vi "Nuclei - sideways pull.vi"() -> ()   [LabVIEW 2010]
uses:
  <vilib>/Utility/error.llb/DialogType.ctl
  <vilib>/DAQmx/read.llb/DAQmx Read (Analog 1D DBL NChan 1Samp).vi
  <vilib>/DAQmx/write.llb/DAQmx Write (Analog DBL 1Chan 1Samp).vi
  <vilib>/DAQmx/read.llb/DAQmx Read (Analog 1D Wfm NChan NSamp).vi
  <vilib>/DAQmx/create/channels.llb/DAQmx Create Channel (AO-Voltage-Basic).vi
  <vilib>/DAQmx/create/channels.llb/DAQmx Create Channel (AI-Voltage-Basic).vi
  <vilib>/DAQmx/configure/timing.llb/DAQmx Timing (Sample Clock).vi
  <vilib>/Utility/inputDevices.llb/keyboardAcquire.vi
  <vilib>/daqmx/miscellaneous.llb/DAQmx Fill In Error Info.vi
  <vilib>/Utility/file.llb/Write To Spreadsheet File (DBL).vi
  Program Files/National Instruments/LabVIEW 2010/resource/objmgr/daqmx.rc
  <vilib>/Analysis/NI_AALBase.lvlib
panel:
  out "element":cluster{dbl[], dbl[]}
  in  "Index #":i32=1
  out "Z Position":dbl
  out "Y Position":dbl
  out "X Position":dbl
  in  "Axial Pulling":T1(tab)=enum."Piezo Move"
  in  "Reset Hysteresis":bool=TRUE
  in  "Axis":u16(ring) items=["X", "Y", "Z"]
  in  "Desired Position (um)":dbl=5.0 min=0.0 max=12.0 format="%0.2f"
  out "X Position":dbl
  out "Y Position":dbl
  out "Z Position":dbl
  in  "Move Piezo":bool=TRUE
  in  "All Axis":bool
  out "Out of Piezo Range":bool
  out "XY Graph":cluster{"Y":dbl[], "Y":dbl[]}[](graph)
  out "# of Samples":i32
  in  "wait time":u32=30
  in  "Speed":dbl=3.0
  in  "stop 3":bool
  out "X Voltage":dbl
  out "XY Graph 2":cluster{dbl[], dbl[]}(graph)
  out "Waveform Graph":dbl[][](graph)
  in  "Desired Frequency 4":dbl=0.01 caption="frequency (Hz)" format="%.2f"
  in  "Save Data":bool=TRUE
  out "?":cluster{dbl[], dbl[]}(graph)
  in  "Axis":u16(ring) items=["X", "Y", "Z"]
  in  "Cycles per Buffer":dbl=1.0 format="%.2f"
  out "Total Time":dbl
  in  "Disp Slope":dbl=-19.0
  in  "Push (nm)":dbl=30.0 min=0.0 max=10.0
  in  "Pull  (nm)":dbl=30.0 min=0.0 max=10.0
  in  "Start":dbl=5.0 min=0.0 max=10.0 format="%#_7g"
  in  "Rate (Hz)":dbl=1000.0 format="%0.2f"
  in  "Manual":bool
  out "?":dbl(graph)
  out "?":dbl(graph)
  in  "Rate":dbl=200.0 caption="Input Rate (Hz)" format="%0.2f"
  in  "Set Point (QPD)":dbl=1.6
  in  "I":dbl=0.001
  in  "P":dbl=0.1
  in  "stop 4":bool caption="stop"
  in  "Axis 2":u16(ring) items=["X", "Y", "Z"]
  in  "Rate 2":dbl=200.0 caption="Input Rate (Hz)" format="%0.2f"
  in  "Axis 3":u16(ring) items=["X", "Y", "Z"]
  out "?":dbl(graph)
  out "?":dbl(graph)
  in  "Set Point (Strain Gauge)":dbl=5.0
  in  "I":dbl=0.001
  in  "P":dbl=0.1
  in  "stop 5":bool caption="stop"
  in  "?":T2(tab)
  in  "maximum volts":dbl=10.0 format="%0.2f"
  in  "minimum volts":dbl=-10.0 format="%0.2f"
  in  "# of Samples":i32=10
  out "?":waveform(dbl)[](graph)
  in  "wait time (ms)":u32=20
  in  "stop 11":bool
  in  "QPD":u16(ring)=1 items=["QPD2", "QPD1"]
  in  "Strain Gauge":bool
  out "?":waveform(dbl)[](graph)
  in  "rate (Hz)":dbl=40000.0 format="%0.2f"
  in  "# Samples  2":i32=120000
  in  "Axis":u16(ring) items=["X", "Y", "Z"]
  out "d":cluster{"Y":dbl[], "Y":dbl[]}[](graph)
  in  "fit end (Hz)":dbl=10000.0
  in  "fit start (Hz)":dbl=30.0
  in  "nbin":dbl=5000.0
  in  "nblock":dbl=100.0
  out "fc error (Hz)  2":dbl
  out "fc (Hz)":dbl
  out "Z (um)":dbl
  in  "# of Measurements":i32=3
  in  "# Samples":i32=50000
  in  "rate (Hz)   2":dbl=50000.0 format="%0.2f"
  in  "stop 2":bool
  in  "Start (um)":dbl format="%0.2f"
  in  "Finish (um)":dbl=4.0 format="%0.2f"
  in  "Step Size (um)":dbl=1.0 format="%0.2f"
  in  "wall":dbl=1.0 format="%0.2f"
  out "Waveform Chart 2":waveform(dbl)[](graph)
  out "?":cluster{"Y":dbl[], "Y":dbl[]}[](graph)
  in  "nbin":dbl=5000.0
  out "?":cluster{"Y":dbl[], "Y":dbl[]}[](graph)
  in  "Amplitude 12":dbl=0.5 caption="Amplitude (um)" format="%0.2p"
  in  "Desired Frequency 5":dbl=0.3 caption="frequency (Hz)" format="%.2f"
  in  "Center (um)":dbl=5.0 format="%0.2p"
  in  "Save Data":bool=TRUE
  in  "Waveform Type 6":T3(ring)=enum."Triangle Wave" caption="Waveform Type"
  in  "Phase":u16(ring)=1 items=["Start", "Middle", "Right End"]
  in  "Axis":u16(ring) items=["X", "Y", "Z"]
  out "?":cluster{"Y":dbl[], "Y":dbl[]}[](graph)
  in  "Axis":u16(ring) items=["X", "Y", "Z"]
  out "Displacement Slope":dbl
  out "?":cluster{"Y":dbl[], "Y":dbl[]}[](graph)
  in  "Phase":u16(ring)=1 items=["Start", "Middle", "Right End"]
  out "X Position 3":dbl
  out "Y Position 3":dbl
  in  "Amplitude 13":dbl=0.5 caption="Amplitude (um)" format="%0.2p"
  in  "Desired Frequency 6":dbl=0.3 caption="frequency (Hz)" format="%.2f"
  in  "Waveform Type 7":T3(ring)=enum."Triangle Wave" caption="Waveform Type"
  in  "Axis":u16(ring) items=["X", "Y", "Z"]
  out "Z Position   3":dbl
  in  "Z start":dbl=5.0 format="%0.2p"
  in  "Z step size":dbl=5.0 format="%0.2p"
  in  "Z finish":dbl=5.0 format="%0.2p"
  in  "Y step size":dbl=5.0 format="%0.2p"
  in  "Y finish":dbl=5.0 format="%0.2p"
  in  "Y start":dbl=5.0 format="%0.2p"
  in  "Filename":string="test"
  # "Run to reset hysteresis!\nPlaces all piezo positions to zero and resets hysteresis parameters\nDo once at the start of the day!"
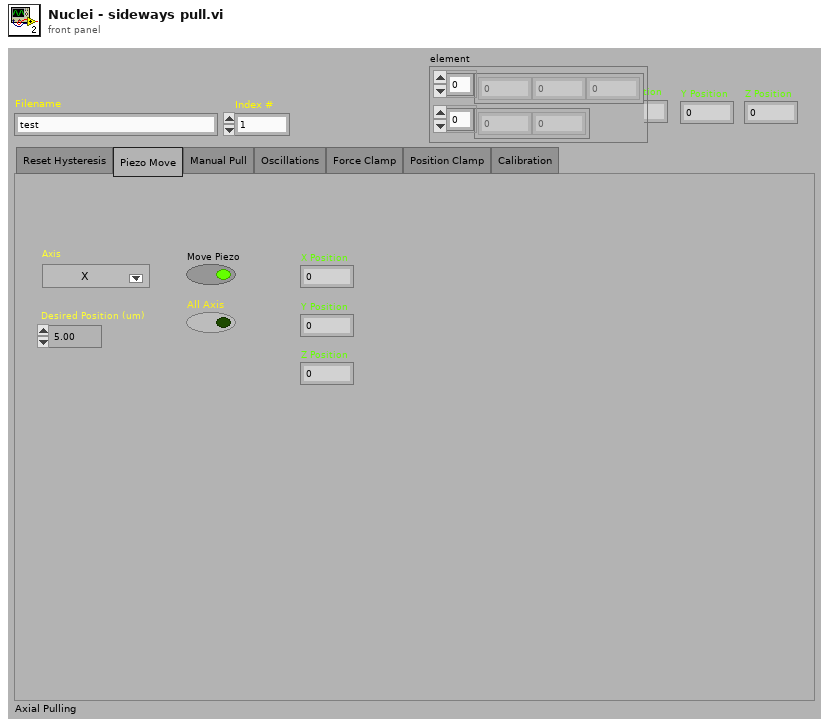
[diagram p1: front panel]
types:
  T1 = enum32{"Reset Hysteresis", "Piezo Move", "Manual Pull", "Oscillations", "Force Clamp", "Position Clamp", "Calibration"}
  T2 = enum32{"QPD", "Power Spectrum", "Axial Step Power Spectrum", "Bead Scan", "Fit Bead Scan", "3D scan"}
  T3 = enum16{"Sine Wave", "Triangle Wave", "Square Wave", "Sawtooth Wave"}
  T4 = enum16{"0", "1", "2", "3", "4", "5", "6", "7", "8", "9", "A", "B", "C", "D", "E", "F", "G", "H", "I", "J", "K", "L", "M", "N", "O", "P", "Q", "R", "S", "T", "U", "V", "W", "X", "Y", "Z", "F1", "F2", "F3", "F4", "F5", "F6", "F7", "F8", "F9", "F10", "F11", "F12", "F13", "F14", "F15", "ADD", "BACK", "BACKSLASH", "CAPITAL", "COMMA", "DECIMAL", "DELETE", "DIVIDE", "DOWN", "END", "EQUALS", "ESCAPE", "GRAVE (`)", "HOME", "INSERT", "LBRACKET", "LCONTROL", "LEFT", "L ALT", "LSHIFT", "LWIN", "MINUS", "MULTIPLY", "NEXT", "NUMLOCK", "NUMPAD_0", "NUMPAD_1", "NUMPAD_2", "NUMPAD_3", "NUMPAD_4", "NUMPAD_5", "NUMPAD_6", "NUMPAD_7", "NUMPAD_8", "NUMPAD_9", "PAUSE", "PERIOD", "PRIOR (PG UP)", "RBRACKET", "RCONTROL", "RETURN", "RIGHT", "R ALT", "RSHIFT", "RWIN", "SCROLL", "SEMICOLON", "SLASH", "SPACE", "SUBTRACT", "TAB", "UP", "ENTER (num pad)", "' (quote)"}[]
  T5 = enum16{"0", "1", "2", "3", "4", "5", "6", "7", "8", "9", "A", "B", "C", "D", "E", "F", "G", "H", "I", "J", "K", "L", "M", "N", "O", "P", "Q", "R", "S", "T", "U", "V", "W", "X", "Y", "Z", "F1", "F2", "F3", "F4", "F5", "F6", "F7", "F8", "F9", "F10", "F11", "F12", "F13", "F14", "F15", "ADD", "BACK", "BACKSLASH", "CAPITAL", "COMMA", "DECIMAL", "DELETE", "DIVIDE", "DOWN", "END", "EQUALS", "ESCAPE", "GRAVE (`)", "HOME", "INSERT", "LBRACKET", "LCONTROL", "LEFT", "L ALT", "LSHIFT", "LWIN", "MINUS", "MULTIPLY", "NEXT", "NUMLOCK", "NUMPAD_0", "NUMPAD_1", "NUMPAD_2", "NUMPAD_3", "NUMPAD_4", "NUMPAD_5", "NUMPAD_6", "NUMPAD_7", "NUMPAD_8", "NUMPAD_9", "PAUSE", "PERIOD", "PRIOR (PG UP)", "RBRACKET", "RCONTROL", "RETURN", "RIGHT", "R ALT", "RSHIFT", "RWIN", "SCROLL", "SEMICOLON", "SLASH", "SPACE", "SUBTRACT", "TAB", "UP", "ENTER (num pad)", "' (quote)"}
  T6 = typedef "DialogType.ctl" = u16
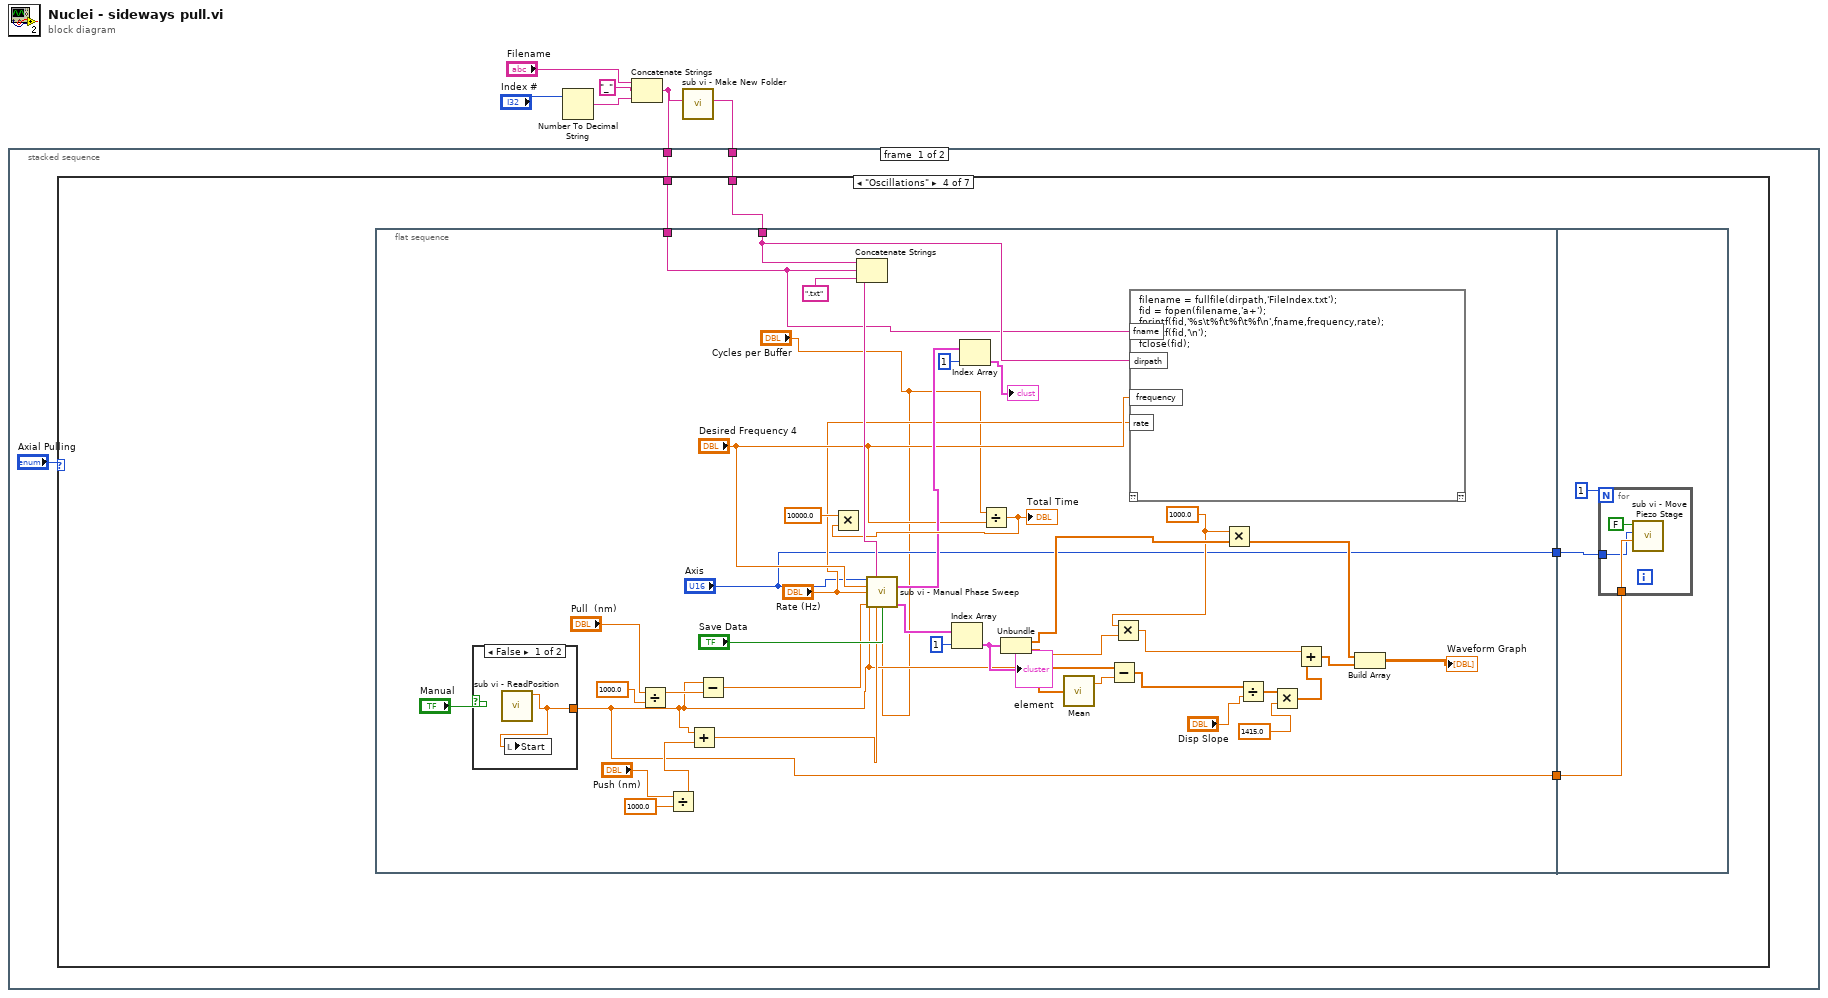
[diagram p0: block diagram]
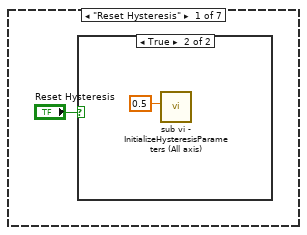
[diagram p2: hidden frame]
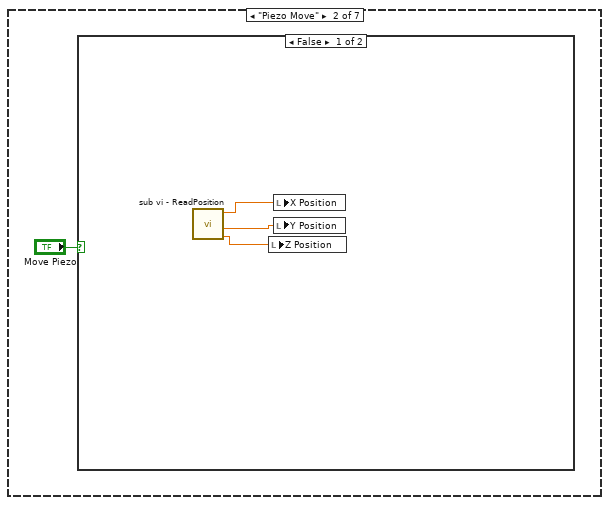
[diagram p4: hidden frame]
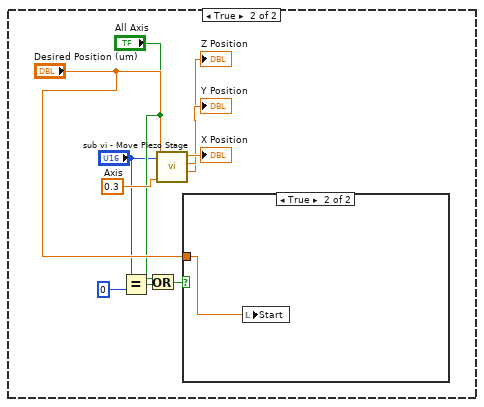
[diagram p5: hidden frame]
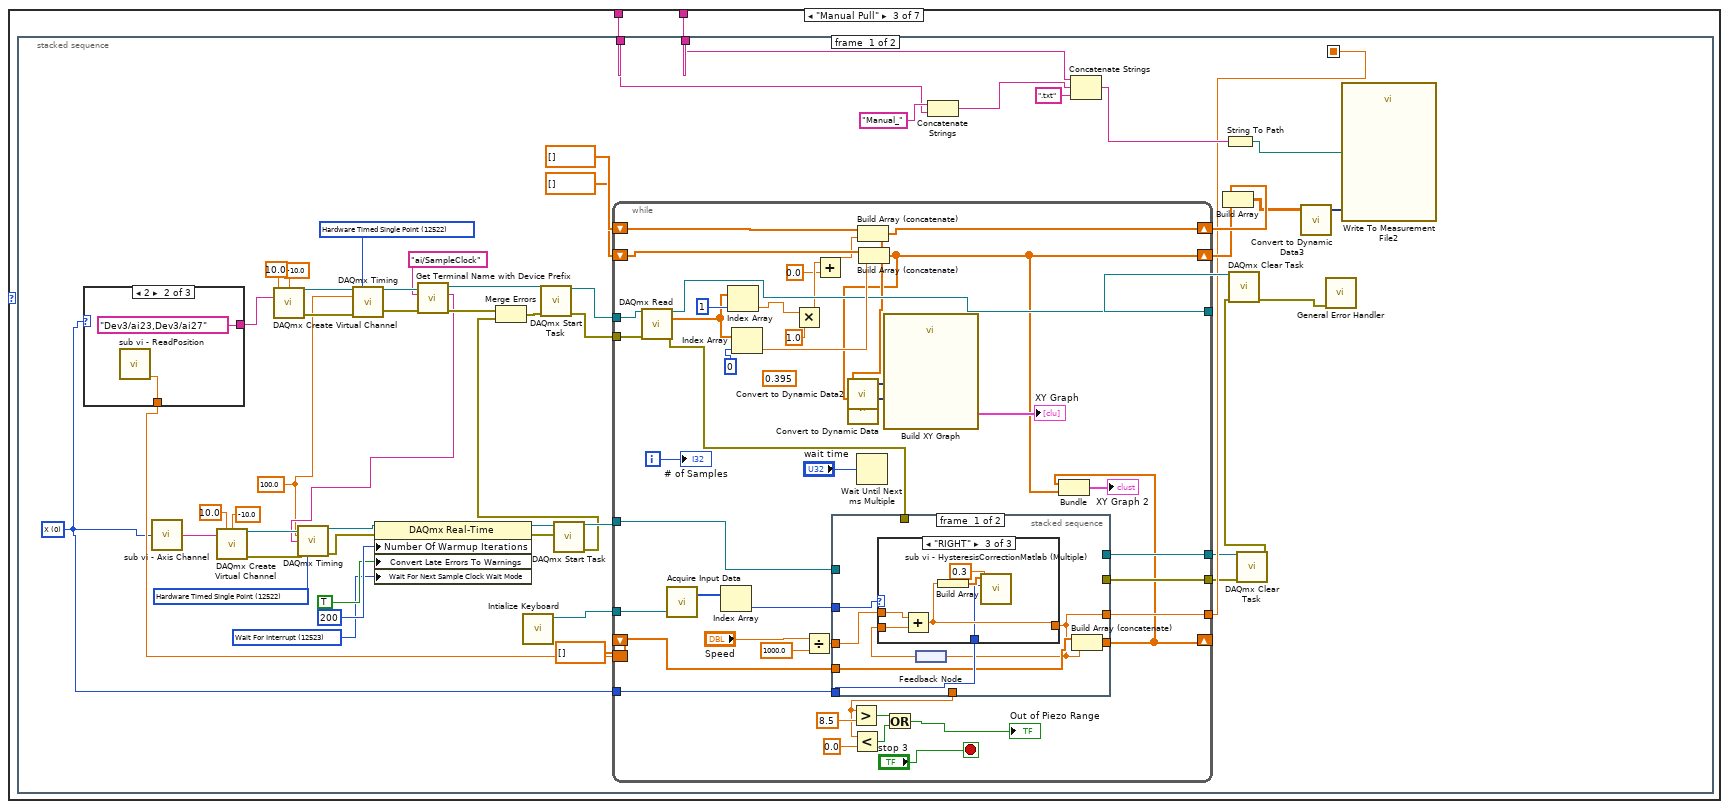
[diagram p7: hidden frame]
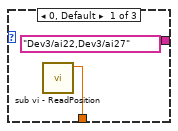
[diagram p8: hidden frame]
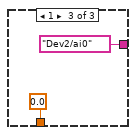
[diagram p9: hidden frame]
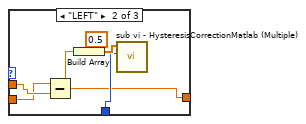
[diagram p11: hidden frame]
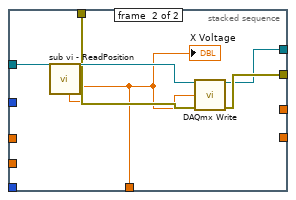
[diagram p12: hidden frame]
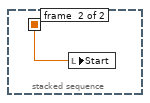
[diagram p13: hidden frame]
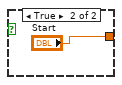
[diagram p14: hidden frame]
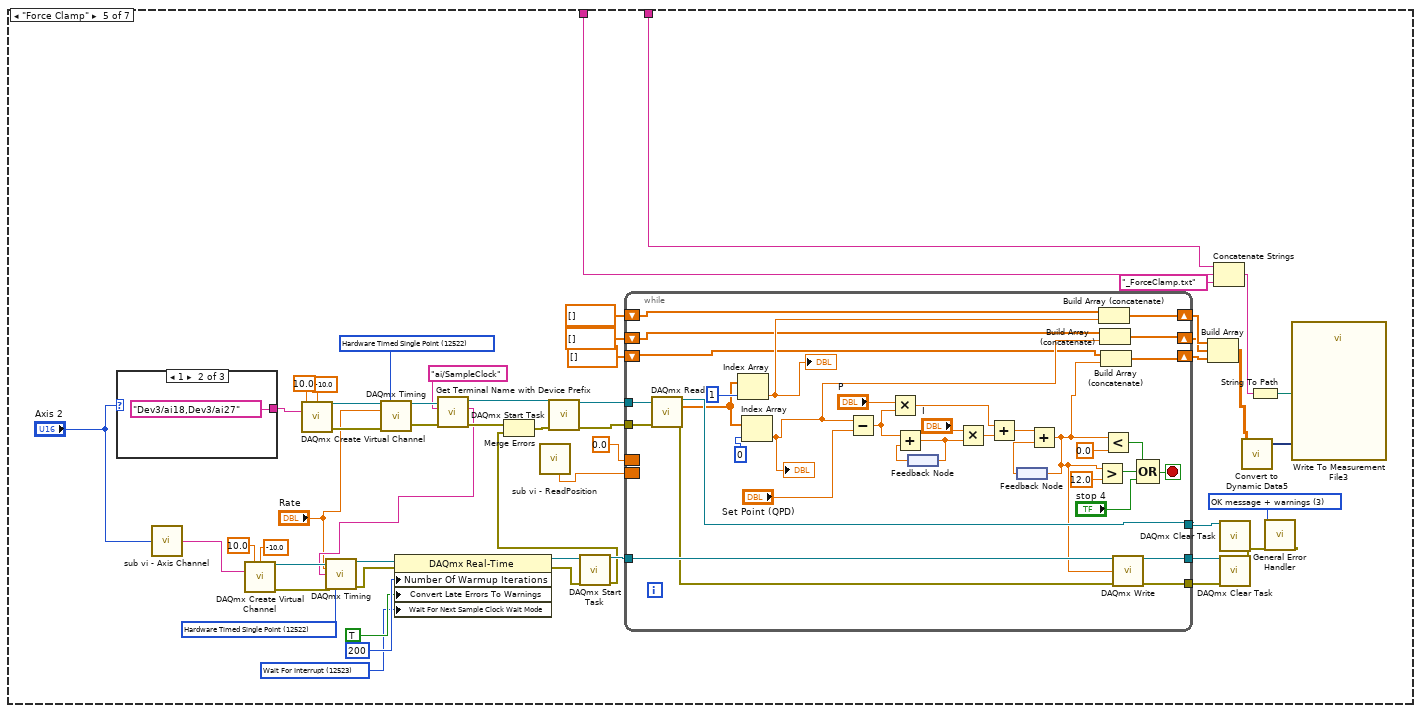
[diagram p15: hidden frame]
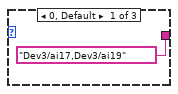
[diagram p16: hidden frame]
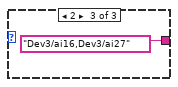
[diagram p17: hidden frame]
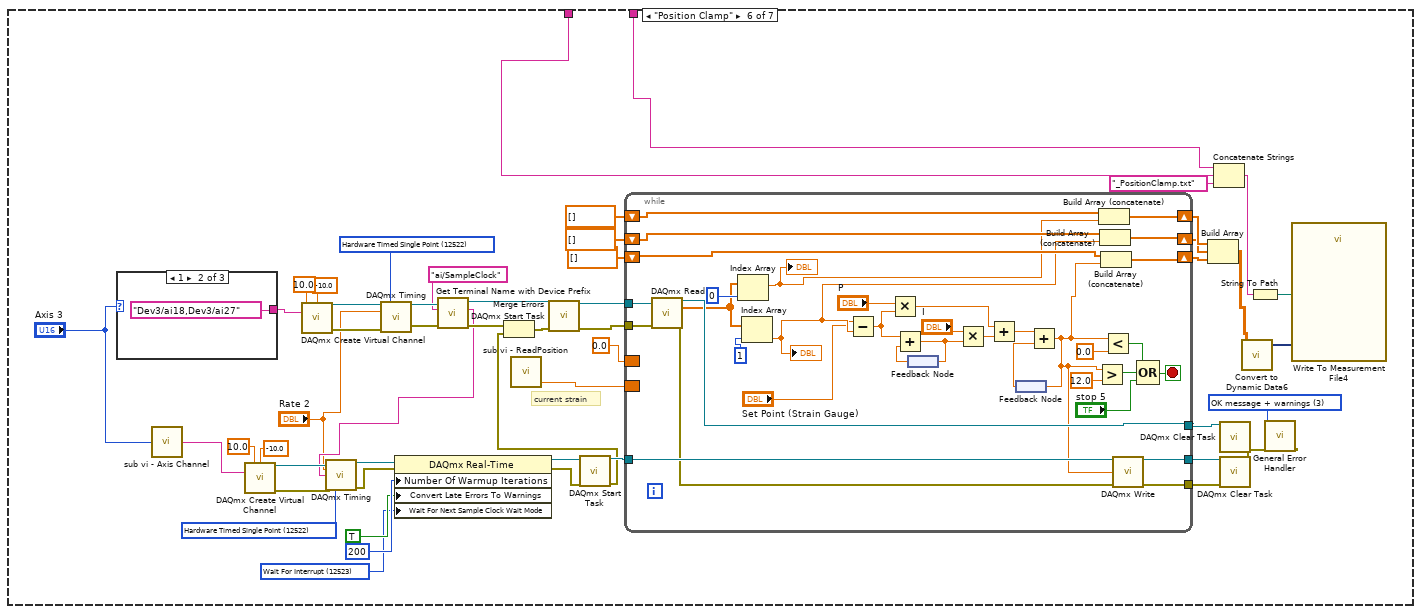
[diagram p18: hidden frame]
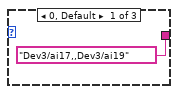
[diagram p19: hidden frame]
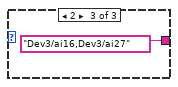
[diagram p20: hidden frame]
diagram:
  n1 = Number To Decimal String(number="Index #") -> (decimal integer string=w3:string)  [unwired: 1 out]
  n2 = Concatenate Strings("Filename", "_" ("string"), w3) -> (w1:string)
  n3 = call "sub vi - Make New Folder.vi"("folder name"=w1) -> ("directory 2"=w2:string)  [unwired: 1 in, 9 out]
  n4 = stacked-sequence {
    tunnel: w2 -> [w8 _]
    tunnel: w1 -> [w7 _]
    frame #0 {
      n5 = case shown="\"Oscillations\"" "Axial Pulling" {
        tunnel: w8 -> [_ _ w28 w160 w213 w301 w392]
        tunnel: w7 -> [_ _ w27 w159 w212 w300 w391]
        frame "Reset Hysteresis" {
          n6 = case shown="True" "Reset Hysteresis" {
            frame False {
            }
            frame True {
              n7 = call "sub vi - InitializeHysteresisParameters (All axis).vi"("frequency"=0.5) -> ()  [unwired: 11 in]
            }
          }
        }
        frame "Piezo Move" {
          n8 = case shown="False" "Move Piezo" {
            frame False {
              n9 = call "sub vi - ReadPosition.vi"() -> ("Z Position"=w13:dbl, "Y Position"=w14:dbl, "X Position"=w15:dbl)  [unwired: 9 out]
              n10 = local write "Z Position"(w13) -> ()
              n11 = local write "X Position"(w15) -> ()
              n12 = local write "Y Position"(w14) -> ()
            }
            frame True {
              n13 = Equal?(x="Axis", y=u16 0) -> (x = y?=w18:bool)
              n14 = Or(x="All Axis", y=w18) -> (x .or. y?=w20:bool)
              n15 = call "sub vi - Move Piezo Stage.vi"("Frequency"=0.3 ("frequency"), "Desired Position (um)"="Desired Position (um)", "Axis"="Axis", "All Axis"="All Axis") -> ("Z Position"=→"Z Position":dbl, "Y Position"=→"Y Position":dbl, "X Position"=→"X Position":dbl)  [unwired: 5 in]
              n16 = case shown="True" w20 {
                tunnel: "Desired Position (um)" -> [_ w26]
                frame False {
                }
                frame True {
                  n17 = local write "Start"(w26) -> ()
                }
              }
            }
          }
        }
        frame "Manual Pull" {
          n18 = stacked-sequence {
            seq-local: [w34 _] -> [_ w156]
            tunnel: w28 -> [w36 _]
            tunnel: w27 -> [w37 _]
            frame #0 {
              w30 = u16 0 items=["X", "Y", "Z"] ("Axis")
              w42 = 100.0 ("rate")
              w63 = 12523 items=["Wait For Interrupt"=12523, "Poll"=12524, "Yield"=12525] ("WaitForNextSampClkWaitMode")
              w76 = 12522 items=["Finite Samples"=10178, "Continuous Samples"=10123, "Hardware Timed Single Point"=12522] ("sample mode")
              w77 = 12522 items=["Finite Samples"=10178, "Continuous Samples"=10123, "Hardware Timed Single Point"=12522] ("sample mode")
              n19 = case shown="2" w30 {
                tunnel: [tag "Dev3/ai22,Dev3/ai27" ("physical channels") tag "Dev3/ai23,Dev3/ai27" ("physical channels") tag "Dev2/ai0" ("physical channels")] -> w58
                tunnel: [w83 w85 0.0 ("Z Position")] -> w43
                frame 0, Default {
                  n20 = call "sub vi - ReadPosition.vi"() -> ("X Position"=w83:dbl)  [unwired: 11 out]
                }
                frame 2 {
                  n21 = call "sub vi - ReadPosition.vi"() -> ("Z Position"=w85:dbl)  [unwired: 11 out]
                }
                frame 1 {
                }
              }
              n22 = call "sub vi - Axis Channel.vi"("Axis"=w30) -> ("physical channels"=w33:tag)
              n23 = call-poly <vilib>:"DAQmx Create Virtual Channel.vi"("maximum value"=10.0, "minimum value"=-10.0, "physical channels"=w33) -> ("task out"=w80:refnum<k21>, "error out"=w79:errorcluster)  [unwired: 6 in, 5 out]
              n24 = call-poly <vilib>:"DAQmx Create Virtual Channel.vi"("maximum value"=10.0, "minimum value"=-10.0, "physical channels"=w58) -> ("task out"=w81:refnum<k21>, "error out"=w82:errorcluster)  [unwired: 6 in, 5 out]
              n25 = call-poly <vilib>:"DAQmx Timing.vi"("task/channels in"=w81, "sample mode"=w77, "rate"=w42, "error in"=w82) -> ("task out"=w75:refnum<k21>, "error out"=w74:errorcluster)  [unwired: 3 in, 7 out]
              n26 = call "Get Terminal Name with Device Prefix.vi"("error in (no error)"=w74, "Local Terminal Name"="ai/SampleClock", "task/channels in"=w75) -> ("error out"=w72:errorcluster, "Terminal Name with Device Prefix"=w71:tag, "task out"=w73:refnum<k21>)  [unwired: 6 out]
              n27 = call-poly <vilib>:"DAQmx Timing.vi"("task/channels in"=w80, "sample mode"=w76, "rate"=w42, "source"=w71, "error in"=w79) -> ("task out"=w68:refnum<k21>, "error out"=w67:errorcluster)  [unwired: 2 in, 7 out]
              n28 = property class="DAQmx Real-Time"(reference=w68, error in=w67, "Number Of Warmup Iterations"=u32 200 ("NumOfWarmupIters"), "Convert Late Errors To Warnings"=TRUE ("ConvLateWarningsToErrors"), "Wait For Next Sample Clock Wait Mode"=w63) -> (reference out=w69:refnum<k21>, error out=w66:errorcluster)
              n29 = call <vilib>:"Intialize Keyboard.vi"() -> ("device ID"=w50:refnum<k1>)  [unwired: 1 in, 10 out]
              n30 = call <vilib>:"DAQmx Start Task.vi"("task/channels in"=w69, "error in"=w66) -> ("task out"=w49:refnum<k21>, "error out"=w45:errorcluster)  [unwired: 12 out]
              n31 = Merge Errors(w72, w45) -> (w78:errorcluster)
              n32 = call <vilib>:"DAQmx Start Task.vi"("task/channels in"=w73, "error in"=w78) -> ("task out"=w56:refnum<k21>, "error out"=w57:errorcluster)  [unwired: 12 out]
              n33 = while {
                tunnel: w57 -> [w125]
                tunnel: w56 -> [w124]
                shift-right: [w115] -> w53
                shift-left: dbl[] [] -> [w90]
                shift-right: [w96] -> w52
                shift-left: dbl[] [] -> [w123]
                tunnel: w50 -> [w121]
                tunnel: w49 -> [w102]
                border: w43 -> [_]
                tunnel: [w120] -> w46
                tunnel: w30 -> [w111]
                tunnel: [w105] -> w34
                tunnel: [w100] -> w32
                tunnel: [w99] -> w31
                shift-right: [w94] -> _
                shift-left: dbl[] [] -> [w95]
                i -> [w117]
                stop <- "stop 3" stop-if-true
                (unwired) 0.395 ("y")
                n34 = call-poly <vilib>:"DAQmx Read.vi"("task/channels in"=w124, "error in"=w125) -> ("task out"=w120:refnum<k21>, "data"=w126:dbl[], "error out"=w101:errorcluster)  [unwired: 1 in, 10 out]
                n35 = call-poly <vilib>:"Acquire Input Data.vi"("device ID"=w121) -> ("keys pressed"=w131:T4)  [unwired: 1 in, 17 out]
                n36 = Index Array(array=w131) -> (element=w129:T5)  [unwired: 1 in]
                n37 = Index Array(array=w126, index=1) -> (element=w110:dbl)
                n38 = Index Array(array=w126, index=0) -> (element=w122:dbl)
                n39 = Multiply(x=w110, y=1.0) -> (x*y=w91:dbl)
                n40 = Divide(x="Speed", y=1000.0) -> (x/y=w112:dbl)
                n41 = Add(x=w91, y=0.0) -> (x+y=w92:dbl)
                n42 = stacked-sequence {
                  tunnel: w129 -> [w138 _]
                  tunnel: w112 -> [w136 _]
                  tunnel: w111 -> [w135 _]
                  tunnel: [w132 _] -> w105
                  tunnel: w102 -> [_ w155]
                  tunnel: w101 -> [_ w154]
                  tunnel: [_ w153] -> w100
                  tunnel: [_ w152] -> w99
                  tunnel: [_ w151] -> w98
                  tunnel: [w134 _] -> w94
                  tunnel: w95 -> [w133 _]
                  frame #0 {
                    n43 = feedback #1() -> (w137:dbl)
                    n44 = case shown="\"RIGHT\"" w138 {
                      tunnel: w136 -> [_ w144 w149]
                      tunnel: w137 -> [w139 w143 w150]
                      tunnel: [w139 w140 w147] -> w132
                      tunnel: w135 -> [_ w141 w146]
                      frame "0", Default {
                      }
                      frame "LEFT" {
                        (unwired) 0.5 ("frequency")
                        n45 = Subtract(x=w143, y=w144) -> (x-y=w140:dbl)
                        n46 = Build Array(w140) -> (w142:dbl[])
                        n47 = call "sub vi - HysteresisCorrectionMatlab (Multiple).vi"("Axis"=w141, "desired positions"=w142) -> ()  [unwired: 8 in, 2 out]
                      }
                      frame "RIGHT" {
                        n48 = Add(x=w149, y=w150) -> (x+y=w147:dbl)
                        n49 = Build Array(w147) -> (w148:dbl[])
                        n50 = call "sub vi - HysteresisCorrectionMatlab (Multiple).vi"("frequency"=0.3, "Axis"=w146, "desired positions"=w148) -> ()  [unwired: 7 in, 2 out]
                      }
                    }
                    n51 = feedback-in #1(w132) -> ()
                    n52 = Build Array (concatenate)(w133, w132) -> (w134:dbl[])
                  }
                  frame #1 {
                    n53 = call "sub vi - ReadPosition.vi"() -> ("X Voltage"=w151:dbl)  [unwired: 11 out]
                    "X Voltage" <- w151
                    n54 = call-poly <vilib>:"DAQmx Write.vi"("task/channels in"=w155, "data"=w151, "error in"=w154) -> ("task out"=w152:refnum<k21>, "error out"=w153:errorcluster)  [unwired: 1 in, 10 out]
                  }
                }
                n55 = Greater?(x=w98, y=8.5) -> (0:w109:bool)
                n56 = Less?(x=w98, y=0.0) -> (x < y?=w108:bool)
                n57 = Wait Until Next ms Multiple(millisecond multiple="wait time") -> ()  [unwired: 1 out]
                n58 = Build Array (concatenate)(w90, w92) -> (w115:dbl[])
                n59 = call "Convert to Dynamic Data2"("Array"=w115) -> ("Dynamic Data Type"=w114:dynamicdata)  [unwired: 3 out]
                n60 = Build Array (concatenate)(w123, w122) -> (w96:dbl[])
                n61 = call "Convert to Dynamic Data"("Array"=w96) -> ("Dynamic Data Type"=w113:dynamicdata)  [unwired: 3 out]
                n62 = call "Build XY Graph"("Y Input"=w113, "X Input"=w114) -> ("XY Graph"=→"XY Graph":cluster{"Y":dbl[], "Y":dbl[]}[])  [unwired: 3 in, 6 out]
                n63 = Or(x=w109, y=w108) -> (x .or. y?=→"Out of Piezo Range":bool)
                n64 = Bundle(w94, w96) -> (→"XY Graph 2":cluster{dbl[], dbl[]})  [unwired: 1 in]
                "# of Samples" <- w117
              }
              n65 = Concatenate Strings("Manual_" ("string"), w37) -> (w38:string)
              n66 = Concatenate Strings(w36, w38, ".txt" ("string")) -> (w41:string)
              n67 = Build Array(w53, w52) -> (w44:dbl[][])
              n68 = String To Path(string=w41) -> (path=w35:path)
              n69 = call <vilib>:"DAQmx Clear Task.vi"("task in"=w31, "error in"=w32) -> ("error out"=w47:errorcluster)  [unwired: 13 out]
              n70 = call <vilib>:"DAQmx Clear Task.vi"("task in"=w46, "error in"=w47) -> ("error out"=w48:errorcluster)  [unwired: 13 out]
              n71 = call "Convert to Dynamic Data3"("2D Array"=w44) -> ("Dynamic Data Type"=w51:dynamicdata)  [unwired: 3 out]
              n72 = call <vilib>:"General Error Handler.vi"("error in (no error)"=w48) -> ()  [unwired: 1 in, 14 out]
              n73 = call "Write To Measurement File2"("Signals"=w51, "Filename"=w35) -> ()  [unwired: 15 in, 3 out]
            }
            frame #1 {
              n74 = local write "Start"(w156) -> ()
            }
          }
        }
        frame "Oscillations" {
          n75 = flat-sequence {
            tunnel: w160 -> [w167]
            tunnel: w159 -> [w166]
            tunnel: ["Axis"] -> w158
            tunnel: [w162] -> w157
            tunnel: w158 -> [w204]
            tunnel: w157 -> [w205]
            frame #0 {
              w173 = 1000.0 ("y")
              n76 = case shown="False" "Manual" {
                tunnel: [w201 "Start"] -> w162
                frame False {
                  n77 = call "sub vi - ReadPosition.vi"() -> ("X Position"=w201:dbl)  [unwired: 6 in, 5 out]
                  n78 = local write "Start"(w201) -> ()
                }
                frame True {
                }
              }
              n79 = Divide(x="Pull  (nm)", y=1000.0) -> (x/y=w183:dbl)
              n80 = Divide(x="Push (nm)", y=1000.0) -> (x/y=w181:dbl)
              n81 = Add(x=w162, y=w181) -> (x+y=w186:dbl)
              n82 = Subtract(x=w162, y=w183) -> (x-y=w184:dbl)
              n83 = Concatenate Strings(w167, w166, ".txt" ("string")) -> (w199:string)
              n84 = call "sub vi - Manual Phase Sweep.vi"("Axis"="Axis", "filename"=w199, "# of Cycles"="Cycles per Buffer", "Desired Frequency"="Desired Frequency 4", "Rate (Hz)"="Rate (Hz)", "Start"=w162, "Low"=w184, "High"=w186, "Save Data"="Save Data") -> ("Displacement vs Position"=w188:cluster{dbl[], dbl[]}[], "Displacement vs Position 2"=w178:cluster{dbl[], dbl[]}[])  [unwired: 2 in, 3 out]
              n85 = Index Array(array=w178, index=1) -> (element=w198:cluster{dbl[], dbl[]})
              "element" <- w198
              n86 = Index Array(array=w188, index=1) -> (element=→"?":cluster{dbl[], dbl[]})
              n87 = Divide(x="Cycles per Buffer", y="Desired Frequency 4") -> (x/y=w190:dbl)
              "Total Time" <- w190
              n88 = Multiply(x=10000.0, y=w190) -> ()  [unwired: 1 out]
              n89 = Unbundle(w198) -> (w174:dbl[], w195:dbl[])
              n90 = call <vilib>:"Mean.vi"("X"=w195) -> ("mean"=w196:dbl)  [unwired: 1 out]
              n91 = Subtract(x=w195, y=w196) -> (x-y=w171:dbl[])
              n92 = Multiply(x=w173, y=w162) -> (x*y=w172:dbl)
              n93 = script code="filename = fullfile(dirpath,'FileIndex.txt');\nfid = fopen(filename,'a+');\nfprintf(fid,'%s\\t%f\\t%f\\t%f\\n',fname,frequency,rate);\nfprintf(fid,'\\n');\nfclose(fid);"("fname"=w166, "dirpath"=w167, "frequency"="Desired Frequency 4", "rate"="Rate (Hz)") -> ()  [unwired: 1 in, 1 out]
              n94 = Multiply(x=w173, y=w174) -> (x*y=w175:dbl[])
              n95 = Divide(x=w171, y="Disp Slope") -> (x/y=w191:dbl[])
              n96 = Multiply(x=w191, y=1415.0) -> (x*y=w170:dbl[])
              n97 = Add(x=w172, y=w170) -> (x+y=w169:dbl[])
              n98 = Build Array(w175, w169) -> (→"Waveform Graph":dbl[][])
            }
            frame #1 {
              n99 = for {
                N: 1 -> [_]
                tunnel: w205 -> [w207]
                tunnel: w204 -> [w206]
                n100 = call "sub vi - Move Piezo Stage.vi"("Desired Position (um)"=w207, "Axis"=w206, "All Axis"=FALSE) -> ()  [unwired: 6 in, 3 out]
              }
            }
          }
        }
        frame "Force Clamp" {
          w234 = 12523 items=["Wait For Interrupt"=12523, "Poll"=12524, "Yield"=12525] ("WaitForNextSampClkWaitMode")
          w249 = 12522 items=["Finite Samples"=10178, "Continuous Samples"=10123, "Hardware Timed Single Point"=12522] ("sample mode")
          w250 = 12522 items=["Finite Samples"=10178, "Continuous Samples"=10123, "Hardware Timed Single Point"=12522] ("sample mode")
          w253 = T6 3 items=["no dialog", "OK message", "continue or stop message", "OK message + warnings", "continue/stop + warnings"] ("type of dialog (OK msg:1)")
          n101 = case shown="1" "Axis 2" {
            tunnel: [tag "Dev3/ai17,Dev3/ai19" ("physical channels") tag "Dev3/ai18,Dev3/ai27" ("physical channels") tag "Dev3/ai16,Dev3/ai27" ("physical channels")] -> w227
            frame 0, Default {
            }
            frame 1 {
            }
            frame 2 {
            }
          }
          n102 = call "sub vi - Axis Channel.vi"("Axis"="Axis 2") -> ("physical channels"=w211:tag)
          n103 = call-poly <vilib>:"DAQmx Create Virtual Channel.vi"("maximum value"=10.0, "minimum value"=-10.0, "physical channels"=w211) -> ("task out"=w256:refnum<k21>, "error out"=w255:errorcluster)  [unwired: 6 in, 5 out]
          n104 = call-poly <vilib>:"DAQmx Create Virtual Channel.vi"("maximum value"=10.0, "minimum value"=-10.0, "physical channels"=w227) -> ("task out"=w257:refnum<k21>, "error out"=w258:errorcluster)  [unwired: 6 in, 5 out]
          n105 = call-poly <vilib>:"DAQmx Timing.vi"("task/channels in"=w257, "sample mode"=w250, "rate"="Rate", "error in"=w258) -> ("task out"=w246:refnum<k21>, "error out"=w245:errorcluster)  [unwired: 3 in, 7 out]
          n106 = call "Get Terminal Name with Device Prefix.vi"("error in (no error)"=w245, "Local Terminal Name"="ai/SampleClock", "task/channels in"=w246) -> ("error out"=w243:errorcluster, "Terminal Name with Device Prefix"=w242:tag, "task out"=w244:refnum<k21>)  [unwired: 6 out]
          n107 = call-poly <vilib>:"DAQmx Timing.vi"("task/channels in"=w256, "sample mode"=w249, "rate"="Rate", "source"=w242, "error in"=w255) -> ("task out"=w239:refnum<k21>, "error out"=w238:errorcluster)  [unwired: 2 in, 7 out]
          n108 = property class="DAQmx Real-Time"(reference=w239, error in=w238, "Number Of Warmup Iterations"=u32 200 ("NumOfWarmupIters"), "Convert Late Errors To Warnings"=TRUE ("ConvLateWarningsToErrors"), "Wait For Next Sample Clock Wait Mode"=w234) -> (reference out=w240:refnum<k21>, error out=w237:errorcluster)
          n109 = call "sub vi - ReadPosition.vi"() -> ("X Voltage"=w209:dbl)  [unwired: 11 out]
          n110 = call <vilib>:"DAQmx Start Task.vi"("task/channels in"=w240, "error in"=w237) -> ("task out"=w254:refnum<k21>, "error out"=w252:errorcluster)  [unwired: 12 out]
          n111 = Merge Errors(w243, w252) -> (w251:errorcluster)
          n112 = call <vilib>:"DAQmx Start Task.vi"("task/channels in"=w244, "error in"=w251) -> ("task out"=w260:refnum<k21>, "error out"=w261:errorcluster)  [unwired: 12 out]
          n113 = while {
            tunnel: w261 -> [w296]
            tunnel: w260 -> [w295]
            tunnel: [w290] -> w259
            tunnel: w254 -> [w294]
            border: w209 -> [_]
            border: 0.0 -> [_]
            tunnel: [w273] -> w226
            tunnel: [w272] -> w225
            shift-right: [w266] -> w217
            shift-left: dbl[] [] -> [w265]
            shift-right: [w267] -> w216
            shift-left: dbl[] [] -> [w264]
            shift-right: [w268] -> w215
            shift-left: dbl[] [] -> [w263]
            stop <- w283 stop-if-true
            n114 = call-poly <vilib>:"DAQmx Read.vi"("task/channels in"=w295, "error in"=w296) -> ("task out"=w290:refnum<k21>, "data"=w279:dbl[], "error out"=w293:errorcluster)  [unwired: 1 in, 10 out]
            n115 = Index Array(array=w279, index=1) -> (element=w269:dbl)
            "?" <- w269
            n116 = Index Array(array=w279, index=0) -> (element=w270:dbl)
            "?" <- w270
            n117 = Subtract(x=w270, y="Set Point (QPD)") -> (x-y=w275:dbl)
            n118 = Multiply(x="P", y=w275) -> (x*y=w286:dbl)
            n119 = feedback #2() -> (w274:dbl)
            n120 = Add(x=w275, y=w274) -> (x+y=w288:dbl)
            n121 = feedback-in #2(w288) -> ()
            n122 = Multiply(x="I", y=w288) -> (x*y=w287:dbl)
            n123 = Add(x=w286, y=w287) -> (x+y=w271:dbl)
            n124 = feedback #3() -> (w289:dbl)
            n125 = Add(x=w271, y=w289) -> (x+y=w262:dbl)
            n126 = feedback-in #3(w262) -> ()
            n127 = Greater?(x=w262, y=12.0) -> (0:w277:bool)
            n128 = Build Array (concatenate)(w265, w269) -> (w266:dbl[])
            n129 = Build Array (concatenate)(w264, w270) -> (w267:dbl[])
            n130 = Build Array (concatenate)(w263, w262) -> (w268:dbl[])
            n131 = Less?(x=w262, y=0.0) -> (x < y?=w278:bool)
            n132 = call-poly <vilib>:"DAQmx Write.vi"("task/channels in"=w294, "data"=w262, "error in"=w293) -> ("task out"=w273:refnum<k21>, "error out"=w272:errorcluster)  [unwired: 1 in, 10 out]
            n133 = Compound Arithmetic op=OR(w278, w277, "stop 4") -> (w283:bool)
          }
          n134 = Build Array(w217, w216, w215) -> (w214:dbl[][])
          n135 = Concatenate Strings(w213, w212, "_ForceClamp.txt" ("string")) -> (w224:string)
          n136 = call <vilib>:"DAQmx Clear Task.vi"("task in"=w226, "error in"=w225) -> ("error out"=w248:errorcluster)  [unwired: 13 out]
          n137 = call <vilib>:"DAQmx Clear Task.vi"("task in"=w259, "error in"=w248) -> ("error out"=w247:errorcluster)  [unwired: 13 out]
          n138 = call "Convert to Dynamic Data5"("2D Array"=w214) -> ("Dynamic Data Type"=w223:dynamicdata)  [unwired: 3 out]
          n139 = String To Path(string=w224) -> (path=w222:path)
          n140 = call <vilib>:"General Error Handler.vi"("type of dialog (OK msg:1)"=w253, "error in (no error)"=w247) -> ()  [unwired: 14 out]
          n141 = call "Write To Measurement File3"("Signals"=w223, "File Name"=w222) -> ()  [unwired: 6 in, 12 out]
        }
        frame "Position Clamp" {
          w325 = 12523 items=["Wait For Interrupt"=12523, "Poll"=12524, "Yield"=12525] ("WaitForNextSampClkWaitMode")
          w340 = 12522 items=["Finite Samples"=10178, "Continuous Samples"=10123, "Hardware Timed Single Point"=12522] ("sample mode")
          w341 = 12522 items=["Finite Samples"=10178, "Continuous Samples"=10123, "Hardware Timed Single Point"=12522] ("sample mode")
          w344 = T6 3 items=["no dialog", "OK message", "continue or stop message", "OK message + warnings", "continue/stop + warnings"] ("type of dialog (OK msg:1)")
          # "current strain"
          n142 = case shown="1" "Axis 3" {
            tunnel: [tag "Dev3/ai17,,Dev3/ai19" ("physical channels") tag "Dev3/ai18,Dev3/ai27" ("physical channels") tag "Dev3/ai16,Dev3/ai27" ("physical channels")] -> w318
            frame 0, Default {
            }
            frame 1 {
            }
            frame 2 {
            }
          }
          n143 = call "sub vi - Axis Channel.vi"("Axis"="Axis 3") -> ("physical channels"=w304:tag)
          n144 = call-poly <vilib>:"DAQmx Create Virtual Channel.vi"("maximum value"=10.0, "minimum value"=-10.0, "physical channels"=w304) -> ("task out"=w347:refnum<k21>, "error out"=w346:errorcluster)  [unwired: 6 in, 5 out]
          n145 = call-poly <vilib>:"DAQmx Create Virtual Channel.vi"("maximum value"=10.0, "minimum value"=-10.0, "physical channels"=w318) -> ("task out"=w348:refnum<k21>, "error out"=w349:errorcluster)  [unwired: 6 in, 5 out]
          n146 = call-poly <vilib>:"DAQmx Timing.vi"("task/channels in"=w348, "sample mode"=w341, "rate"="Rate 2", "error in"=w349) -> ("task out"=w337:refnum<k21>, "error out"=w336:errorcluster)  [unwired: 3 in, 7 out]
          n147 = call "Get Terminal Name with Device Prefix.vi"("error in (no error)"=w336, "Local Terminal Name"="ai/SampleClock", "task/channels in"=w337) -> ("error out"=w334:errorcluster, "Terminal Name with Device Prefix"=w333:tag, "task out"=w335:refnum<k21>)  [unwired: 6 out]
          n148 = call-poly <vilib>:"DAQmx Timing.vi"("task/channels in"=w347, "sample mode"=w340, "rate"="Rate 2", "source"=w333, "error in"=w346) -> ("task out"=w330:refnum<k21>, "error out"=w329:errorcluster)  [unwired: 2 in, 7 out]
          n149 = property class="DAQmx Real-Time"(reference=w330, error in=w329, "Number Of Warmup Iterations"=u32 200 ("NumOfWarmupIters"), "Convert Late Errors To Warnings"=TRUE ("ConvLateWarningsToErrors"), "Wait For Next Sample Clock Wait Mode"=w325) -> (reference out=w331:refnum<k21>, error out=w328:errorcluster)
          n150 = call "sub vi - ReadPosition.vi"() -> ("X Voltage"=w302:dbl)  [unwired: 11 out]
          n151 = call <vilib>:"DAQmx Start Task.vi"("task/channels in"=w331, "error in"=w328) -> ("task out"=w345:refnum<k21>, "error out"=w343:errorcluster)  [unwired: 12 out]
          n152 = Merge Errors(w334, w343) -> (w342:errorcluster)
          n153 = call <vilib>:"DAQmx Start Task.vi"("task/channels in"=w335, "error in"=w342) -> ("task out"=w351:refnum<k21>, "error out"=w352:errorcluster)  [unwired: 12 out]
          n154 = while {
            tunnel: w352 -> [w387]
            tunnel: w351 -> [w386]
            tunnel: [w381] -> w350
            tunnel: w345 -> [w385]
            border: w302 -> [_]
            border: 0.0 -> [_]
            tunnel: [w365] -> w317
            tunnel: [w364] -> w316
            shift-right: [w360] -> w308
            shift-left: dbl[] [] -> [w359]
            shift-right: [w361] -> w307
            shift-left: dbl[] [] -> [w358]
            shift-right: [w362] -> w306
            shift-left: dbl[] [] -> [w357]
            stop <- w374 stop-if-true
            n155 = call-poly <vilib>:"DAQmx Read.vi"("task/channels in"=w386, "error in"=w387) -> ("task out"=w381:refnum<k21>, "data"=w371:dbl[], "error out"=w384:errorcluster)  [unwired: 1 in, 10 out]
            n156 = Index Array(array=w371, index=0) -> (element=w355:dbl)
            "?" <- w355
            n157 = Index Array(array=w371, index=1) -> (element=w354:dbl)
            "?" <- w354
            n158 = Subtract(x="Set Point (Strain Gauge)", y=w354) -> (x-y=w367:dbl)
            n159 = Multiply(x="P", y=w367) -> (x*y=w377:dbl)
            n160 = feedback #4() -> (w366:dbl)
            n161 = Add(x=w367, y=w366) -> (x+y=w379:dbl)
            n162 = feedback-in #4(w379) -> ()
            n163 = Multiply(x="I", y=w379) -> (x*y=w378:dbl)
            n164 = Add(x=w377, y=w378) -> (x+y=w363:dbl)
            n165 = feedback #5() -> (w380:dbl)
            n166 = Add(x=w363, y=w380) -> (x+y=w356:dbl)
            n167 = feedback-in #5(w356) -> ()
            n168 = Greater?(x=w356, y=12.0) -> (0:w369:bool)
            n169 = Build Array (concatenate)(w359, w355) -> (w360:dbl[])
            n170 = Build Array (concatenate)(w358, w354) -> (w361:dbl[])
            n171 = Build Array (concatenate)(w357, w356) -> (w362:dbl[])
            n172 = Less?(x=w356, y=0.0) -> (x < y?=w370:bool)
            n173 = call-poly <vilib>:"DAQmx Write.vi"("task/channels in"=w385, "data"=w356, "error in"=w384) -> ("task out"=w365:refnum<k21>, "error out"=w364:errorcluster)  [unwired: 1 in, 10 out]
            n174 = Compound Arithmetic op=OR(w370, w369, "stop 5") -> (w374:bool)
          }
          n175 = Build Array(w308, w307, w306) -> (w305:dbl[][])
          n176 = Concatenate Strings(w301, w300, "_PositionClamp.txt" ("string")) -> (w315:string)
          n177 = call <vilib>:"DAQmx Clear Task.vi"("task in"=w317, "error in"=w316) -> ("error out"=w339:errorcluster)  [unwired: 13 out]
          n178 = call <vilib>:"DAQmx Clear Task.vi"("task in"=w350, "error in"=w339) -> ("error out"=w338:errorcluster)  [unwired: 13 out]
          n179 = call "Convert to Dynamic Data6"("2D Array"=w305) -> ("Dynamic Data Type"=w314:dynamicdata)  [unwired: 3 out]
          n180 = String To Path(string=w315) -> (path=w313:path)
          n181 = call <vilib>:"General Error Handler.vi"("type of dialog (OK msg:1)"=w344, "error in (no error)"=w338) -> ()  [unwired: 14 out]
          n182 = call "Write To Measurement File4"("Signals"=w314, "File Name"=w313) -> ()  [unwired: 6 in, 12 out]
        }
        frame "Calibration" {
          n183 = case shown="\"Axial Step Power Spectrum\"" "?" {
            tunnel: w392 -> [_ w424 w443 w450 w512 w580]
            tunnel: w391 -> [_ w423 _ w449 w511 w579]
            frame "QPD" {
              n184 = case shown="1" "QPD" {
                tunnel: [w411 w412] -> w399
                tunnel: "Strain Gauge" -> [w410 _]
                frame 0, Default {
                  n185 = call "sub vi - QPD channels 2.vi"("Include Position?"=w410) -> ("QPD Channels"=w411:tag)  [unwired: 9 out]
                }
                frame 1 {
                  n186 = call "sub vi - QPD channels.vi"() -> ("QPD Channels"=w412:tag)  [unwired: 11 out]
                }
              }
              n187 = case shown="False" "Strain Gauge" {
                tunnel: [w408 w409] -> w397
                frame False {
                  w408 = 10106 items=["default"=-1, "RSE"=10083, "NRSE"=10078, "Differential"=10106, "Pseudodifferential"=12529] ("input terminal configuration")
                }
                frame True {
                  w409 = -1 items=["default"=-1, "RSE"=10083, "NRSE"=10078, "Differential"=10106, "Pseudodifferential"=12529] ("input terminal configuration")
                }
              }
              n188 = call-poly <vilib>:"DAQmx Create Virtual Channel.vi"("maximum value"="maximum volts", "minimum value"="minimum volts", "input terminal configuration"=w397, "physical channels"=w399, "name to assign"="QPD") -> ("task out"=w396:refnum<k21>, "error out"=w395:errorcluster)  [unwired: 4 in, 5 out]
              n189 = call <vilib>:"DAQmx Start Task.vi"("task/channels in"=w396, "error in"=w395) -> ("task out"=w403:refnum<k21>, "error out"=w402:errorcluster)  [unwired: 12 out]
              n190 = while {
                shift-right: [w418] -> w405
                shift-left: w403 -> [w420]
                shift-right: [w417] -> w404
                shift-left: w402 -> [w419]
                stop <- "stop 11" stop-if-true
                n191 = Wait Until Next ms Multiple(millisecond multiple="wait time (ms)") -> ()  [unwired: 1 out]
                n192 = call-poly <vilib>:"DAQmx Read.vi"("task/channels in"=w420, "number of samples per channel"="# of Samples", "error in"=w419) -> ("task out"=w418:refnum<k21>, "data"=→"?":waveform(dbl)[], "error out"=w417:errorcluster)  [unwired: 10 out]
              }
              n193 = call <vilib>:"DAQmx Clear Task.vi"("task in"=w405, "error in"=w404) -> ("error out"=w406:errorcluster)  [unwired: 13 out]
              n194 = call <vilib>:"General Error Handler.vi"("error in (no error)"=w406) -> ()  [unwired: 2 in, 13 out]
            }
            frame "Bead Scan" {
              n195 = Concatenate Strings(w424, w423, "StuckBead.txt" ("string")) -> (w427:string)
              n196 = call "QPD - Pizeo Calibration (Single sweep) 2.vi"("Axis"="Axis", "Waveform Type"="Waveform Type 6", "Rate (Hz)"=500.0, "Center"="Center (um)", "Amplitude"="Amplitude 12", "Desired Frequency"="Desired Frequency 5", "Phase"="Phase", "Cycles per Buffer"=1.0, "Save Data"="Save Data", "filename"=w427) -> ("Displacement vs Position 2"=→"?":cluster{dbl[], dbl[]}[])  [unwired: 2 in, 7 out]
            }
            frame "Fit Bead Scan" {
              n197 = script code="[filename dirpath] = uigetfile(fullfile(dirpath,'*.txt'),'Select displacement slope file');\n\ndata = dlmread(fullfile(dirpath,filename));\n\nswitch(axis)\ncase 0\n   index = 3;\ncase 1\n   index = 4;\ncase 2\n   index = 2;\notherwise\n   index = 3;\nend\n\npos = data(:,1);\nstrain = data(:,5);\nqpd = data(:,index);\n\nfigure(1); clf;\nplot(strain,qpd);\n[x y button] = ginput(2);\n\nrange = find(strain > min(x) & strain < max(x));\n\nqpd2 = qpd(range);\nstrain2 = strain(range);\npos2 = pos(range);\n\nf = fittype('a*x+b');\n[c gof] = fit(strain2,qpd2,f,'startpoint',[1 1]);\n\nfitqpd = c(strain2);\n\nqpd2 = qpd2';\nstrain2 = strain2';\npos2 = pos2';\nfitqpd2 = fitqpd';\n\nslope = c.a;\nclose all;"("dirpath"=w443, "axis"="Axis") -> ("qpd2"=w441:dbl[], "strain2"=w440:dbl[], "fitqpd2"=w439:dbl[], "slope"=→"Displacement Slope":dbl)  [unwired: 1 in, 2 out]
              n198 = Bundle(w440, w439) -> (w437:cluster{dbl[], dbl[]})  [unwired: 1 in]
              n199 = Bundle(w440, w441) -> (w438:cluster{dbl[], dbl[]})  [unwired: 1 in]
              n200 = Build Array(w438, w437) -> (→"?":cluster{dbl[], dbl[]}[])
            }
            frame "3D scan" {
              n201 = Subtract(x="Z finish", y="Z start") -> (x-y=w448:dbl)
              n202 = Divide(x=w448, y="Z step size") -> (x/y=w446:dbl)
              n203 = for {
                N: w446 -> [_]
                tunnel: w450 -> [w463]
                tunnel: w449 -> [w462]
                tunnel: "Z start" -> [w461]
                tunnel: "Z step size" -> [w459]
                i -> [w452]
                n204 = Multiply(x=w459, y=w452) -> (x*y=w460:dbl)
                n205 = Add(x=w461, y=w460) -> (x+y=w453:dbl)
                n206 = Subtract(x="Y finish", y="Y start") -> (x-y=w457:dbl)
                n207 = Divide(x=w457, y="Y step size") -> (x/y=w456:dbl)
                n208 = Number To Decimal String(number=w452) -> (decimal integer string=w451:string)  [unwired: 1 in]
                n209 = stacked-sequence {
                  tunnel: w463 -> [_ w477]
                  tunnel: w462 -> [_ w476]
                  tunnel: w456 -> [_ w475]
                  tunnel: "Y start" -> [_ w474]
                  tunnel: "Y step size" -> [_ w473]
                  tunnel: w453 -> [w464 _]
                  tunnel: w451 -> [_ w472]
                  frame #0 {
                    w468 = u16 2 items=["X", "Y", "Z"] ("Axis")
                    n210 = call "sub vi - Move Piezo Stage.vi"("stop"=TRUE, "Frequency"=0.3 ("frequency"), "Desired Position (um)"=w464, "Axis"=w468, "All Axis"=FALSE) -> ("Z Position"=→"Z Position   3":dbl, "Y Position"=→"Y Position 3":dbl, "X Position"=→"X Position 3":dbl)  [unwired: 4 in]
                  }
                  frame #1 {
                    n211 = for {
                      N: w475 -> [_]
                      tunnel: w477 -> [w486]
                      tunnel: w476 -> [w485]
                      tunnel: w474 -> [w484]
                      tunnel: w473 -> [w483]
                      tunnel: w472 -> [w479]
                      i -> [w480]
                      n212 = Multiply(x=w483, y=w480) -> (x*y=w482:dbl)
                      n213 = Add(x=w484, y=w482) -> (x+y=w481:dbl)
                      n214 = Number To Decimal String(number=w480) -> (decimal integer string=w478:string)  [unwired: 1 in]
                      n215 = stacked-sequence {
                        tunnel: w486 -> [_ w502]
                        tunnel: w485 -> [_ w501]
                        tunnel: w481 -> [w490 _]
                        tunnel: w479 -> [_ w498]
                        tunnel: w478 -> [_ w496]
                        frame #0 {
                          w491 = u16 1 items=["X", "Y", "Z"] ("Axis")
                          n216 = call "sub vi - Move Piezo Stage.vi"("stop"=TRUE, "Frequency"=0.3 ("frequency"), "Desired Position (um)"=w490, "Axis"=w491, "All Axis"=FALSE) -> ("Z Position"=w487:dbl, "Y Position"=w488:dbl, "X Position"=w489:dbl)  [unwired: 4 in]
                          n217 = local write "Z Position   3"(w487) -> ()
                          n218 = local write "Y Position 3"(w488) -> ()
                          n219 = local write "X Position 3"(w489) -> ()
                        }
                        frame #1 {
                          n220 = Concatenate Strings(w502, w501, "scan_z=" ("string"), w498, "_y=" ("string"), w496, ".txt" ("string")) -> (w500:string)
                          n221 = call "QPD - Pizeo Calibration (Single sweep) 2.vi"("Axis"="Axis", "Waveform Type"="Waveform Type 7", "Rate (Hz)"=500.0, "Amplitude"="Amplitude 13", "Desired Frequency"="Desired Frequency 6", "Phase"="Phase", "Save Data"=TRUE, "filename"=w500) -> ("Displacement vs Position 2"=→"?":cluster{dbl[], dbl[]}[])  [unwired: 4 in, 7 out]
                        }
                      }
                    }
                  }
                }
              }
            }
            frame "Power Spectrum", Default {
              n222 = flat-sequence {
                tunnel: w511 -> [w518]
                tunnel: w512 -> [w517]
                tunnel: [w516] -> w514
                tunnel: [w515] -> w513
                tunnel: w514 -> [w529]
                tunnel: w513 -> [w524]
                frame #0 {
                  w522 = u16 1 items=["QPD2", "QPD1"] ("Axis  2")
                  n223 = call "sub vi - PowerSpectrum 2.vi"("number of samples per channel"="# Samples  2", "rate (Hz)"="rate (Hz)", "Save Raw Data"=FALSE, "Axis  2"=w522) -> (3:w516:waveform(dbl)[])  [unwired: 1 in, 6 out]
                  "?" <- w516
                  n224 = Concatenate Strings(w517, w518, "PowerSpectrum.txt" ("string")) -> (w515:string)
                }
                frame #1 {
                  n225 = Two Button Dialog(message="Would you like to fit this?", 1:"no" ("F button name (\"Cancel\")"), 2:"yes" ("T button name (\"OK\")")) -> (T button?=w531:bool)
                  n226 = case shown="2" "Axis" {
                    tunnel: w529 -> [w536 w540 w544]
                    tunnel: [w535 w539 w543] -> w528
                    frame 0, Default {
                      n227 = Index Array(array=w536, index=2) -> (element=w538:waveform(dbl))
                      n228 = Unbundle By Name(w538) -> ("Y"=w535:dbl[])
                    }
                    frame 1 {
                      n229 = Index Array(array=w540, index=3) -> (element=w542:waveform(dbl))
                      n230 = Unbundle By Name(w542) -> ("Y"=w539:dbl[])
                    }
                    frame 2 {
                      n231 = Index Array(array=w544, index=1) -> (element=w546:waveform(dbl))
                      n232 = Unbundle By Name(w546) -> ("Y"=w543:dbl[])
                    }
                  }
                  n233 = case shown="True" w531 {
                    tunnel: "Axis" -> [_ w565]
                    tunnel: w528 -> [w554 w564]
                    tunnel: [w547 w560] -> w526
                    frame False {
                      n234 = local read "rate (Hz)"() -> (w551:dbl)
                      n235 = local read "nbin"() -> (w555:dbl)
                      n236 = script code="sampling_f = rate;\nfNyq = sampling_f/2;\ndelta_t = 1/sampling_f;\nX = X - mean(X);\nnumX = length(X);\ntime = (0:numX-1)'*delta_t;\nT = time(end);\nf = ((1:numX)/T)';\n\nFT = delta_t*fft(X);\nP = FT.*conj(FT)/T;\n\n% Block power spectrum\n[f2  P] = BinPowerSpectrum(f,P,nbin);\n\nind = find(f2 < fNyq,1,'last'); \nf2 = f2(1:ind)';\nP = P(1:ind)';\nf2 = f2(2:end);\nP = P(2:end);"("rate"=w551, "X"=w554, "nbin"=w555) -> ("f2"=w549:dbl[], "P"=w548:dbl[])  [unwired: 1 in, 1 out]
                      n237 = Bundle(w549, w548) -> (w550:cluster{dbl[], dbl[]})  [unwired: 1 out]
                      n238 = Build Array(w549, w548) -> (w547:dbl[][])
                      n239 = Build Array(cluster{dbl[], dbl[]} {[], []} ("element"), w550) -> (w553:cluster{dbl[], dbl[]}[])
                      n240 = local write "d"(w553) -> ()
                    }
                    frame True {
                      n241 = local read "rate (Hz)"() -> (w563:dbl)
                      n242 = script code="close all;\n\nhydroparam.filter = 0;\nhydroparam.l = 0;\nhydroparam.R = 0.56e-6;\nhydroparam.nu = 1.33e-3;\n\nif A == 0\n axis = 2;\nelseif A == 1\naxis = 3;\nelseif A == 2\naxis = 1;\nend\naxisname = 'ZXY';\nX = X';\n% calculate power spectrum\n[f P T fNyq] = CalculatePowerSpectrum(X,sampling_f);\n\n% Block power spectrum\n[fb_plot Pb_plot] = BinPowerSpectrum(f,P,nbin);\n\n% Block Power Spectrum\n[fb Pb s nblock_plot] = BlockPowerSpectrum(f,P,nblock);\n\n%  Choose data to be fit \nind = find(fb > Lfit_start & fb <= Lfit_end);\nxfin = fb(ind);\nyfin = Pb(ind);\nsfin = s(ind);\n\n% initial guess of power spectrum fit\np0 = FitInitialGuess(f,P,fNyq); \n\n %  Fit Power Spectrum to Lorentzian    \n[parameters sigma_par cv chi2] = FitPowerSpectrum(xfin,yfin,sfin,p0,hydroparam,fNyq);\n\n% calculate fitted curve\nPfit = theoreticalP(parameters,fb,fNyq,hydroparam);\n\nfc = parameters(1); \nfcerror = sigma_par(1);\n\nfb_plot = fb_plot';\nPb_plot = Pb_plot';\nfb = fb';\nPfit = Pfit';\nf = f';\nP = P';"("A"=w565, "sampling_f"=w563, "nblock"="nblock", "nbin"="nbin", "Lfit_start"="fit start (Hz)", "Lfit_end"="fit end (Hz)", "X"=w564) -> ("fc"=→"fc (Hz)":dbl, "fcerror"=→"fc error (Hz)  2":dbl, "fb_plot"=w557:dbl[], "Pb_plot"=w556:dbl[], "Pfit"=w558:dbl[], "fb"=w559:dbl[])  [unwired: 4 out]
                      n243 = Build Array(w559, w558, w557, w556) -> (w560:dbl[][])
                      n244 = Bundle(w557, w556) -> (w566:cluster{dbl[], dbl[]})  [unwired: 1 out]
                      n245 = Bundle(w559, w558) -> (w561:cluster{dbl[], dbl[]})  [unwired: 1 out]
                      n246 = Build Array(w561, w566) -> (→"d":cluster{dbl[], dbl[]}[])
                    }
                  }
                  n247 = String To Path(string=w524) -> (path=w527:path)
                  n248 = call "Convert to Dynamic Data7"("2D Array"=w526) -> ("Dynamic Data Type"=w525:dynamicdata)  [unwired: 3 in]
                  n249 = call "Write To Measurement File5"("Signals"=w525, "Filename"=w527) -> ()  [unwired: 15 in, 3 out]
                }
              }
            }
            frame "Axial Step Power Spectrum" {
              # "Step in Z-axis and take power spectrum"
              n250 = while {
                tunnel: "Start (um)" -> [w601]
                tunnel: "Finish (um)" -> [w602]
                tunnel: "Step Size (um)" -> [w599]
                shift-right: [w592] -> w575
                shift-left: dbl[] [] -> [w591]
                tunnel: w580 -> [w590]
                tunnel: w579 -> [w589]
                tunnel: [w588] -> w577 mode=indexing
                i -> [w594]
                stop <- w595 stop-if-true
                n251 = Subtract(x=w602, y=w601) -> (x-y=w600:dbl)
                n252 = Divide(x=w600, y=w599) -> (x/y=w598:dbl)
                n253 = Less?(x=w598, y=w594) -> (x < y?=w597:bool)
                n254 = Number To Decimal String(number=w594) -> (decimal integer string=w593:string)  [unwired: 1 out]
                n255 = stacked-sequence {
                  seq-local: [_ _ w618 _] -> [_ _ _ w644]
                  seq-local: [_ _ w617 _] -> [_ _ _ w645]
                  tunnel: w601 -> [w607 _ _ _]
                  tunnel: w599 -> [w608 _ _ _]
                  tunnel: w594 -> [w609 _ _ _]
                  tunnel: w593 -> [_ _ w621 _]
                  tunnel: [_ w614 _ _] -> w592
                  tunnel: w591 -> [_ w612 _ _]
                  tunnel: w590 -> [_ _ w620 _]
                  tunnel: w589 -> [_ _ w619 _]
                  tunnel: [w603 _ _ _] -> w588
                  frame #0 {
                    w610 = u16 2 items=["X", "Y", "Z"] ("Axis")
                    # "Step in Z-axis"
                    n256 = Multiply(x=w608, y=w609) -> (x*y=w606:dbl)
                    n257 = Add(x=w607, y=w606) -> (x+y=w605:dbl)
                    n258 = call "sub vi - Move Piezo Stage (Single).vi"("frequency"=0.5, "Desired Position (um)"=w605, "Axis"=w610) -> ("Z Position"=w603:dbl)  [unwired: 2 out]
                    "Z (um)" <- w603
                  }
                  frame #1 {
                    n259 = call "sub vi - Strain Gauge Single.vi"("rate"=500.0, "# of Samples"=500, "Strain Gauge"=tag "Dev2/ai27") -> ("mean"=w613:dbl)  [unwired: 1 in, 7 out]
                    n260 = Build Array (concatenate)(w612, w613) -> (w614:dbl[])
                  }
                  frame #2 {
                    # "Power Spectrum"
                    n261 = for {
                      N: "# of Measurements" -> [_]
                      tunnel: w621 -> [w642]
                      tunnel: w620 -> [w637]
                      tunnel: w619 -> [w636]
                      tunnel: [w626] -> w618
                      tunnel: [w625] -> w617
                      i -> [w638]
                      w631 = u16 0 items=["QPD2", "QPD1"] ("Axis  2")
                      n262 = Number To Decimal String(number=w638) -> (decimal integer string=w639:string)  [unwired: 1 out]
                      n263 = Concatenate Strings(w637, w636, w642, "_" ("string"), w639, ".txt" ("string")) -> (w632:string)
                      n264 = call "sub vi - PowerSpectrum 2.vi"("filename"=w632, "number of samples per channel"="# Samples", "rate (Hz)"="rate (Hz)   2", "Save Raw Data"=TRUE, "Axis  2"=w631) -> (3:w627:waveform(dbl)[])  [unwired: 6 out]
                      n265 = Index Array(array=w627, index=1) -> (element=w624:waveform(dbl))
                      n266 = Index Array(array=w627, index=0) -> (element=w628:waveform(dbl))
                      n267 = Build Array(w628, w624) -> (→"Waveform Chart 2":waveform(dbl)[])
                      n268 = Unbundle By Name(w624) -> ("Y"=w625:dbl[])
                      n269 = Unbundle By Name(w628) -> ("Y"=w626:dbl[])
                    }
                  }
                  frame #3 {
                    n270 = local read "rate (Hz)   2"() -> (w643:dbl)
                    n271 = script code="close all;\n\nhydroparam.filter = 0;\nhydroparam.l = 0;\nhydroparam.R = 0.56e-6;\nhydroparam.nu = 1.33e-3;\n\n% calculate power spectrum\n[f P T fNyq] = CalculatePowerSpectrum(X,sampling_f);\n[fb_plot Pb_plot] = BinPowerSpectrum(f,P,nbin);\nfb_plot = fb_plot';\nPb_plot = Pb_plot';\n\n[f P T fNyq] = CalculatePowerSpectrum(Z,sampling_f);\n[fb_plot2 Pb_plot2] = BinPowerSpectrum(f,P,nbin);\nfb_plot2 = fb_plot2';\nPb_plot2 = Pb_plot2';"("nbin"="nbin", "X"=w645, "Z"=w644, "sampling_f"=w643) -> ("fb_plot"=w649:dbl[], "Pb_plot"=w648:dbl[], "fb_plot2"=w651:dbl[], "Pb_plot2"=w652:dbl[])  [unwired: 2 out]
                    n272 = Bundle(w649, w648) -> (w650:cluster{dbl[], dbl[]})  [unwired: 1 out]
                    n273 = Bundle(w651, w652) -> (w653:cluster{dbl[], dbl[]})  [unwired: 1 out]
                    n274 = Build Array(w650, w653) -> (→"?":cluster{dbl[], dbl[]}[])
                  }
                }
                n275 = Or(x=w597, y="stop 2") -> (x .or. y?=w595:bool)
              }
              n276 = Concatenate Strings(w580, w579, "_axial_Position.txt" ("string")) -> (w582:string)
              n277 = Build Array (concatenate)("wall", w577) -> (w576:dbl[])
              n278 = String To Path(string=w582) -> (path=w581:path)
              n279 = Build Array(w576, w575) -> (w574:dbl[][])
              n280 = Transpose 2D Array(2D array=w574) -> (transposed array=w573:dbl[][])
              n281 = call-poly <vilib>:"Write To Spreadsheet File.vi"("2D data"=w573, "file path (dialog if empty)"=w581) -> ()  [unwired: 4 in, 3 out]
            }
          }
        }
      }
    }
    frame #1 {
      n282 = call "sub vi - ReadPosition.vi"() -> ("Z Position"=→"Z Position":dbl, "Y Position"=→"Y Position":dbl, "X Position"=→"X Position":dbl)  [unwired: 9 out]
    }
  }
